vi "Get package_templatemessage.vi"(8 "error in (no error)":errorcluster, 11 "gRPCid":T1) -> (0 "error out":errorcluster, 2 "package_templatemessage":T2, 3 "gRPCid out":T1)   [LabVIEW 2019, in "Generated_server.lvlib"]
uses:
  Generated_server.lvlib
  package_templatemessage.ctl
  <vilib>/gRPC/LabVIEW gRPC Library/Shared/grpcId.ctl
  2ed25e12-861d-4677-8ead-ace2906b2041.vi
  c750bf2f-d32b-4a25-a00a-5db67bc240fd.vi
  <vilib>/gRPC/LabVIEW gRPC Library/Shared/TranslateGrpcError.vi
  <vilib>/gRPC/LabVIEW gRPC Library/Server API/Server/Get Server DLL Path.vi
  <vilib>/Utility/error.llb/Error Cluster From Error Code.vi
  <vilib>/Utility/error.llb/Simple Error Handler.vi
  <vilib>/gRPC/LabVIEW gRPC Library/grpc-lvsupport-release.lvlib
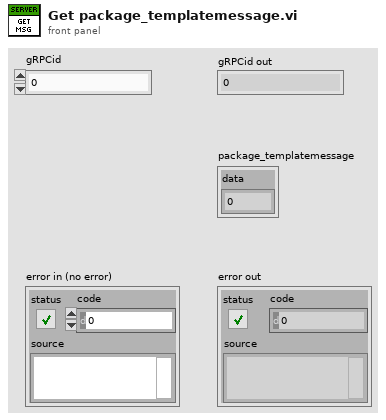
[diagram p1: front panel]
types:
  T1 = typedef "grpc-lvsupport-release.lvlib/grpcId.ctl" = u64
  T2 = typedef "Generated_server.lvlib/package_templatemessage.ctl" = cluster{"data":sgl}
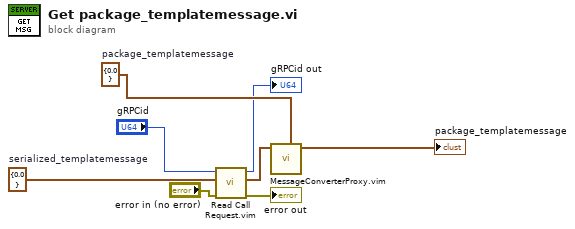
[diagram p0: block diagram]
diagram:
  w6 = T2 {"data"=0.0}  # serialized_templatemessage
  w5 = T2 {"data"=0.0}  # package_templatemessage
  n1 = call "Read Call Request.vim"("error in"="error in (no error)", "Request Type"=w6, "gRPCid in"="gRPCid") -> ("error out"=→"error out":errorcluster, "Request Data"=w4:T2, "gRPCid out"=→"gRPCid out":T1)  [unwired: 6 in]
  n2 = call "MessageConverterProxy.vim"("package_templatemessage_type"=w5, "serialized_templatemessage"=w4) -> ("package_templatemessage"=→"package_templatemessage":T2)  [unwired: 9 in]
